vi "SS_observer.vi"(7 "y(k)":sgl format="%#_13g", 9 "X":sgl[](array[numeric])=[0.0, 0.0, 0.0, 0.0, 0.0, 0.0, 0.0, 0.0, 0.0, 0.0, 0.0, 0.0, 0.0, 0.0, 0.0, 0.0, 0.0, 0.0, 0.0, 0.0, 0.0, 0.0, 0.0, 0.0, 0.0], 10 "u(k)":sgl format="%#_13g", 11 "NS":i16) -> (3 "Ax + Bu + Lye":sgl[](array[numeric]))   [LabVIEW 2017]
uses:
  <vilib>/Platform/TimedLoop/XDataNode/timing_clust.ctl
  <vilib>/Platform/TimedLoop/XDataNode/nitl_modes.ctl
  <vilib>/Platform/TimedLoop/XDataNode/wakeup.ctl
  <vilib>/rvi/Emulation/niFpgaSctlEmulationGetInTimedLoop.vi
  <vilib>/rvi/Emulation/niFpgaEmulationReportErrorSimple.vi
  <vilib>/rvi/Emulation/niFpgaGetClockAttributes.vi
  <vilib>/rvi/Emulation/niFpgaCriticalErrorInLSC.vi
  <vilib>/Platform/TimedLoop/XDataNode/XDataNode.xnode
  <vilib>/Platform/TimedLoop/XDataNode/XDNodeRunTimeDep.lvlib
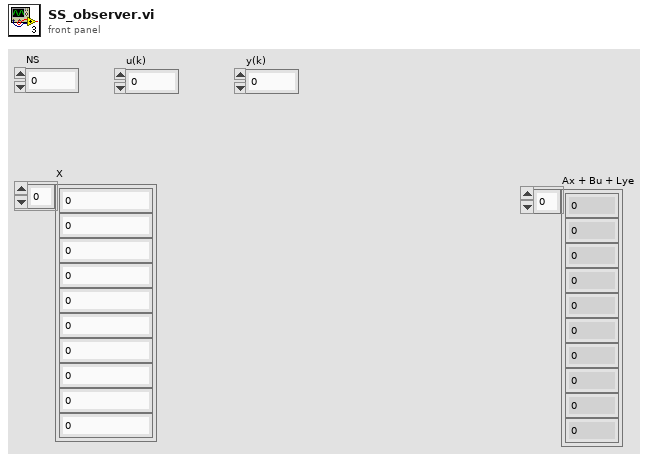
[diagram p1: front panel]
types:
  T1 = typedef "XDNodeRunTimeDep.lvlib/timing_clust.ctl" = cluster{"Expected End [f-1]":u64, "Actual End [f-1]":u64, "Finished Late? [f-1]":bool, "Expected End [i-1]":u64, "Actual End [i-1]":u64, "Finished Late? [i-1]":bool, "Expected Start [i]":u64, "Actual Start [i]":u64, "Expected Start [f]":u64, "Actual Start [f]":u64, "Source Name":string, "Structure Name":string, "Period":i64, "Deadline":i64, "Offset":i64, "Start":i64, "Priority":i32, "Timeout":i32, "Mode":T2, "Wakeup Reason":T3, "Error":errorcluster, "Source Type":string, "Secondary Source Type":string, "Global End Time":u64, "Global Start Time":u64, "Frame Duration":u64, "Iteration Duration":u64, "Assigned CPU":i32, "I/O Scan Engine Mode":u32}
  T2 = typedef "XDNodeRunTimeDep.lvlib/nitl_modes.ctl" = enum32{"No Change", "Process missed periods, maintain original phase", "Discard missed periods, maintain original phase", "Process missed periods, ignore original phase", "Discard missed periods, ignore original phase"}
  T3 = typedef "XDNodeRunTimeDep.lvlib/wakeup.ctl" = enum32{"Normal", "Aborted", "Asynchronous wakeup", "Timing source error", "Timed loop error", "Timeout"}
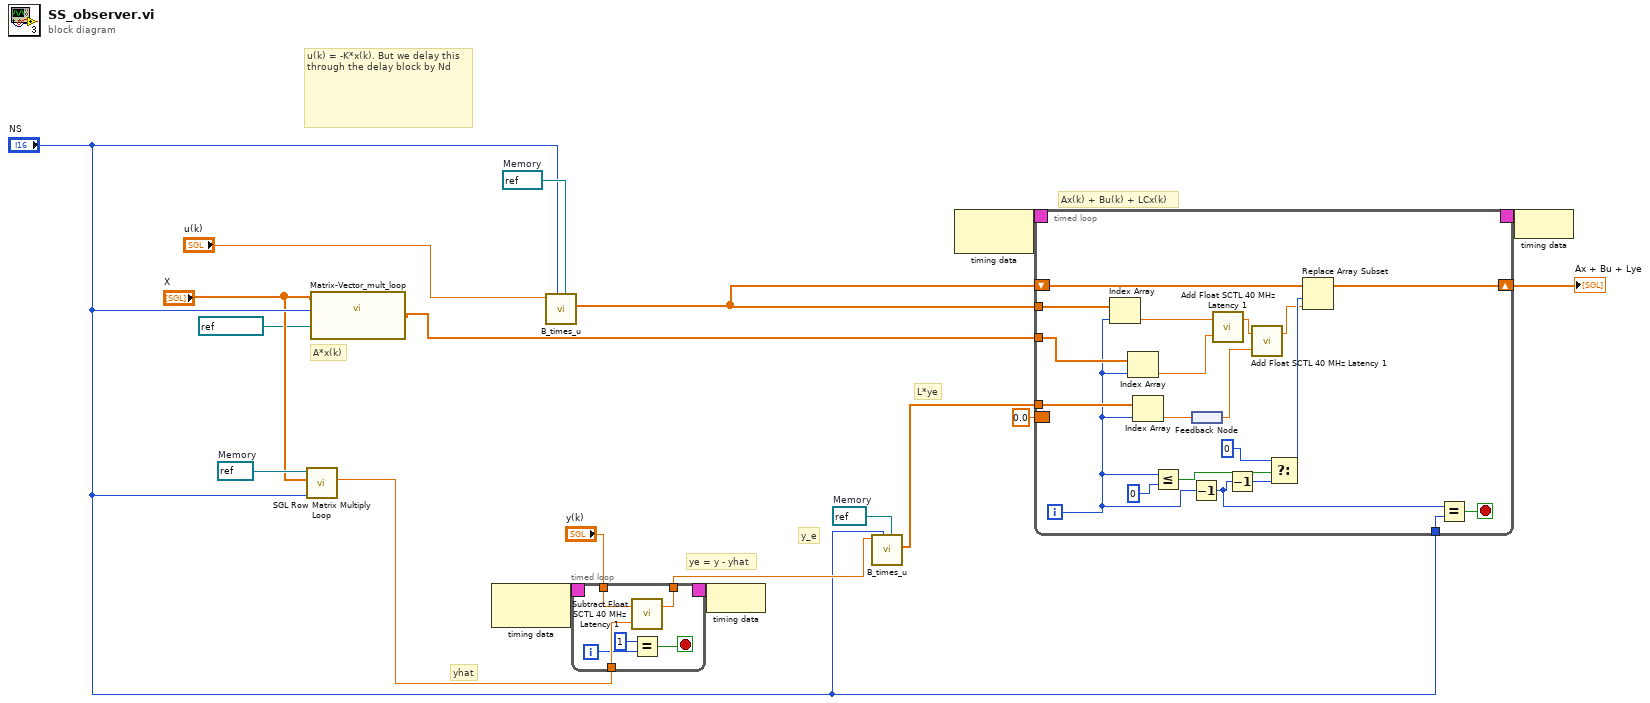
[diagram p0: block diagram]
diagram:
  w13 = refnum<k21> "L"  # Memory
  w12 = refnum<k21> "C"  # Memory
  w11 = refnum<k21> "Bz"  # Memory
  # "ye = y - yhat"
  # "yhat"
  # "A*x(k)"
  # "L*ye"
  # "y_e"
  # "u(k) = -K*x(k). But we delay this through the delay block by Nd"
  # "Ax(k) + Bu(k) + LCx(k)"
  n1 = call "SGL Row Matrix Multiply Loop.vi"("NS"="NS", "X"="X", "Refnum in"=w12) -> ("Numeric"=w9:sgl)  [unwired: 8 in]
  n2 = call "Matrix-Vector_mult_loop.vi"("Row"=refnum<k21> "AasCol", "Ns"="NS", "X"="X") -> ("A x X"=w5:sgl[])  [unwired: 8 in]
  n3 = node-c288() -> (w17:T1)  [unwired: 1 in]
  n4 = call "B_times_u.vi"("Memory"=w11, "NS"="NS", "u"="u(k)") -> ("product(vector)"=w6:sgl[])  [unwired: 8 in]
  n5 = timed-loop {
    timing: w17 -> [_]
    timing-out: [_] -> w16
    tunnel: [w25] -> w7
    tunnel: "y(k)" -> [w24]
    tunnel: w9 -> [w23]
    i -> [w21]
    stop <- w22 stop-if-true
    n6 = call "Subtract Float SCTL 40 MHz Latency 1.vi"("y"=w23, "x"=w24) -> ("x[k-1]-y[k-1]"=w25:sgl)  [unwired: 1 out]
    n7 = Equal?(x=i16 1, y=w21) -> (x = y?=w22:bool)
  }
  n8 = node-c288(w16) -> ()
  n9 = call "B_times_u.vi"("Memory"=w13, "NS"="NS", "u"=w7) -> ("product(vector)"=w8:sgl[])  [unwired: 8 in]
  n10 = node-c288() -> (w19:T1)  [unwired: 1 in]
  n11 = timed-loop {
    timing: w19 -> [_]
    timing-out: [_] -> w18
    tunnel: w6 -> [w45]
    tunnel: w5 -> [w46]
    tunnel: "NS" -> [w41]
    shift-right: [w44] -> w10
    shift-left: w6 -> [w43]
    tunnel: w8 -> [w38]
    border: sgl 0.0 -> [_]
    i -> [w34]
    stop <- w47 stop-if-true
    n12 = Index Array(array=w45, index=w34) -> (element=w40:sgl)
    n13 = Index Array(array=w46, index=w34) -> (element=w39:sgl)
    n14 = Index Array(array=w38, index=w34) -> (element=w36:sgl)
    n15 = Less Or Equal?(x=w34, y=i16 0) -> (x <= y?=w33:bool)
    n16 = Decrement(x=w34) -> (x-1=w29:i32)
    n17 = feedback #1() -> (w32:sgl)
    n18 = feedback-in #1(w36) -> ()
    n19 = call "Add Float SCTL 40 MHz Latency 1.vi"("y"=w39, "x"=w40) -> ("x[k-1]+y[k-1]"=w31:sgl)  [unwired: 1 out]
    n20 = Decrement(x=w29) -> (x-1=w28:i32)
    n21 = call "Add Float SCTL 40 MHz Latency 1.vi"("y"=w32, "x"=w31) -> ("x[k-1]+y[k-1]"=w30:sgl)  [unwired: 1 out]
    n22 = Select(t=i16 0, s=w33, f=w28) -> (s? t:f=w42:i32)
    n23 = Replace Array Subset(array=w43, new element=w30, index=w42) -> (w44:sgl[])
    n24 = Equal?(x=w29, y=w41) -> (x = y?=w47:bool)
  }
  "Ax + Bu + Lye" <- w10
  n25 = node-c288(w18) -> ()
